vi "Flow_Status_Cluster_images.vi"() -> ()   [LabVIEW 2016]
panel:
  out "Flow_status_cluster":T1
  # "N2 Flow Low"
  # "N2 Off"
  # "N2 Flow ok"
  # "H2 Flow Low"
  # "CO Flow Low"
  # "CO2 Flow Low"
  # "CO2 Off"
  # "CO Off"
  # "H2 Off"
  # "H2 Flow ok"
  # "CO Flow ok"
  # "CO2 Flow ok"
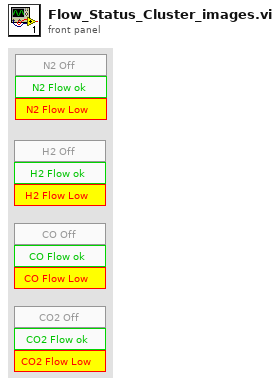
[diagram p1: front panel]
types:
  T1 = cluster{"N2_Flow_state 2":u16, "N2_Flow_state 3":u16, "N2_Flow_state 4":u16, "N2_Flow_state 5":u16}
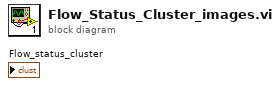
[diagram p0: block diagram]
diagram:
